vi "Panel Init Dry Flow Meter.vi"(11 "Error In":errorcluster) -> (6 "Heat Val.":dbl, 8 "BTUF3":string[][](array[string]), 15 "Error Out":errorcluster)   [LabVIEW 2012]
panel:
  in  "Gas Type":string(combo)="Natural Gas"
  in  "lower limit":dbl=500.0
  in  "upper limit":dbl=5000.0
  in  "stop":bool
  in  "Todays Calorimeter Reading":string
  # "BTU/ft3"
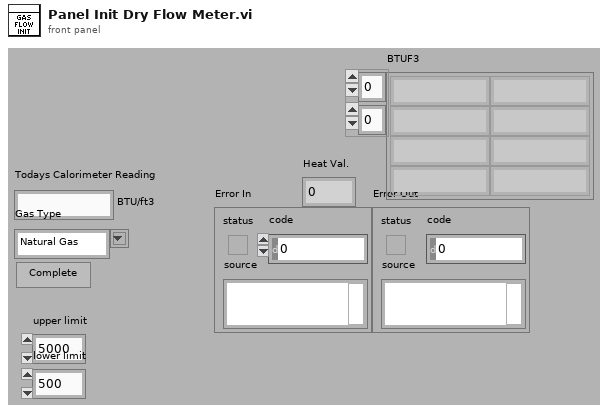
[diagram p1: front panel]
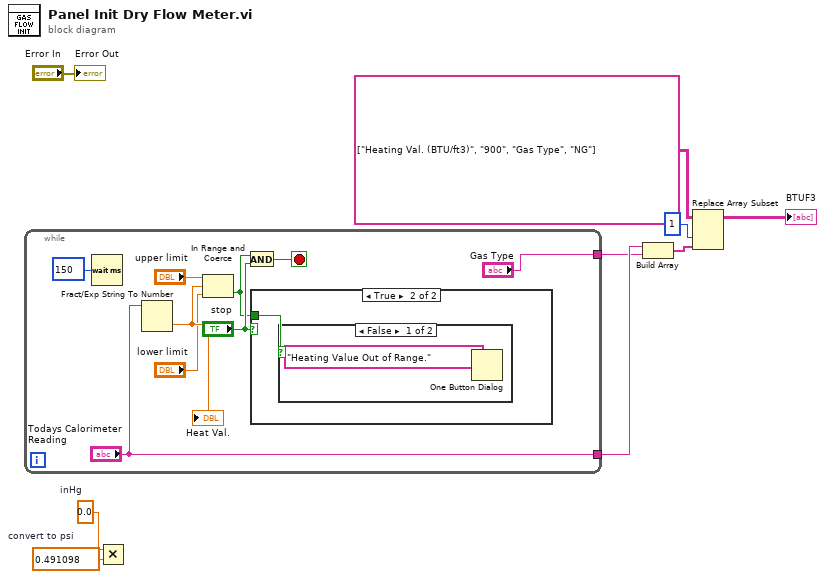
[diagram p0: block diagram]
diagram:
  w3 = 0.0  # inHg
  w8 = 0.491098  # convert to psi
  n1 = while {
    tunnel: ["Todays Calorimeter Reading"] -> w5
    tunnel: ["Gas Type"] -> w2
    stop <- w13 stop-if-true
    n2 = Wait (ms)(milliseconds to wait=u32 150) -> ()  [unwired: 1 out]
    n3 = Fract/Exp String To Number(string="Todays Calorimeter Reading") -> (number=w16:dbl)  [unwired: 3 in, 1 out]
    "Heat Val." <- w16
    n4 = In Range and Coerce(upper limit="upper limit", x=w16, lower limit="lower limit") -> (In Range?=w11:bool)  [unwired: 1 out]
    n5 = And(x=w11, y="stop") -> (x .and. y?=w13:bool)
    n6 = case shown="True" "stop" {
      tunnel: w11 -> [_ w19]
      frame False {
      }
      frame True {
        n7 = case shown="False" w19 {
          frame False {
            n8 = One Button Dialog(message="Heating Value Out of Range.") -> ()  [unwired: 1 in, 1 out]
          }
          frame True {
          }
        }
      }
    }
  }
  n9 = Multiply(x=w3, y=w8) -> ()  [unwired: 1 out]
  n10 = Build Array(w5, w2) -> (w4:string[])
  n11 = Replace Array Subset(array=string[][] [["Heating Val. (BTU/ft3)", "900"], ["Gas Type", "NG"]] ("appended array"), new element=w4, index (col)=1 ("disabled index (col)")) -> (→"BTUF3":string[][])  [unwired: 1 in]
  "Error Out" <- "Error In"
